vi "ROSTerminal.vi"() -> ()   [LabVIEW 2012]
doc: "Provides a space to debug any errors in code by:\n-allowing for testing connection to master\n-showing open nodes\n-linking to a website for viewing what is passed back and forth on a topic\n-linking to a website for the master to view what is passed back and forth\n-showing open logs\n-providing IP for you and Master"
uses:
  <userlib>/ROSforLV/ROS/Code/SubVIs/_ROSControl.ctl
  <userlib>/ROSforLV/ROS/Code/SubVIs/_ROSDirection.ctl
  <userlib>/ROSforLV/ROS/Code/_ROSDefinition.vi
  <vilib>/Platform/browser.llb/Open URL in Default Browser (string).vi
panel:
  out "elements":string[](array[string])
  in  "CloseServers":bool
  in  "Servers":i32(listbox)
  in  "Open HTML":bool
  in  "CloseNodes":bool
  in  "Nodes":i32(listbox)
  in  "ClearOldLogs":bool
  in  "Logs":i32(listbox)
  in  "OpenNodes":bool
  in  "MasterWeb":bool
  in  "MyWeb":bool
  in  "StartMaster":bool
  in  "UDP":bool
  out "My IP":string="http://192.168.1.8"
  in  "Done":bool
  out "Live":bool
  in  "Test":bool
  in  "Current Master":string="192.168.1.110:11311"
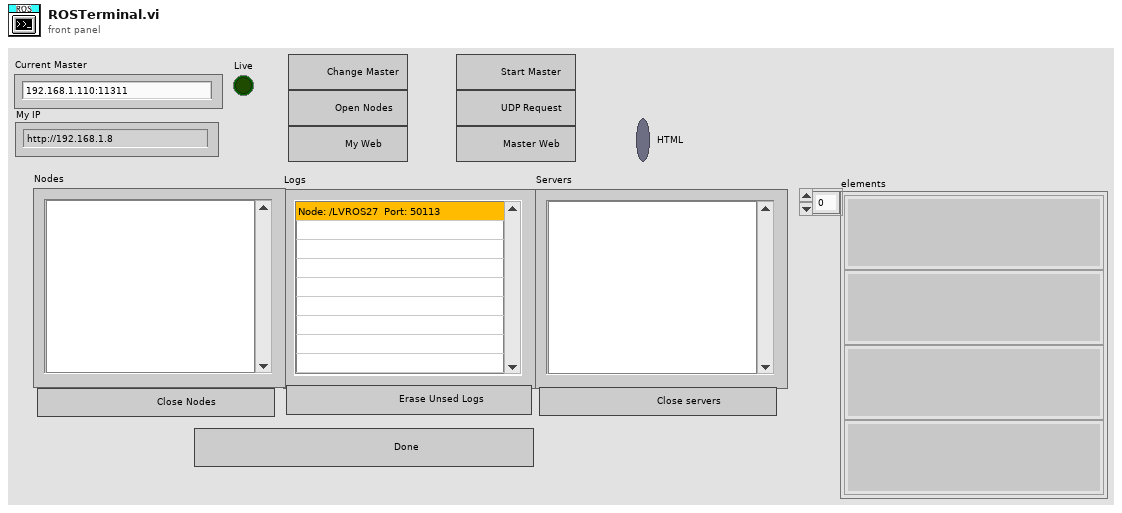
[diagram p1: front panel]
types:
  T1 = typedef "_ROSControl.ctl" = cluster{"topic port":u16, "Node":string, "topic":string, "type":string, "node port":u16, "error ":errorcluster, "Direction":T2, "Update (ms)":u16, "FIFO size":u16}
  T2 = typedef "_ROSDirection.ctl" = enum16{"Node", "Publisher", "Subscriber", "ServiceClient", "ServiceProvider"}
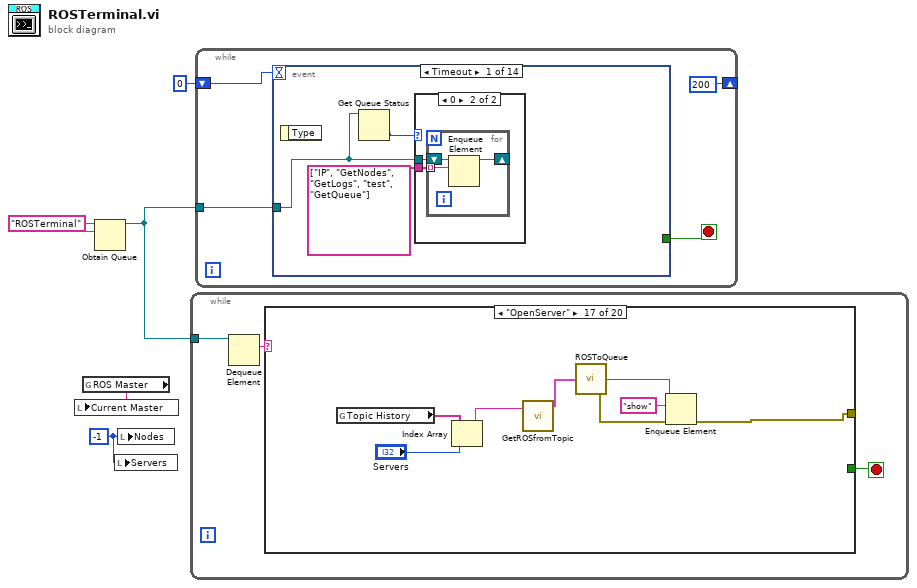
[diagram p0: block diagram]
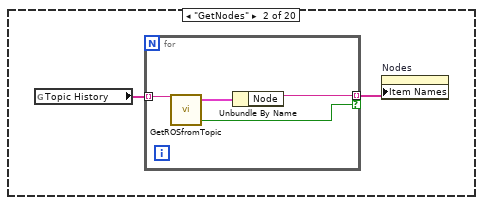
[diagram p3: hidden frame]
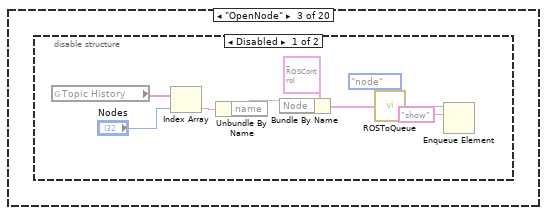
[diagram p4: hidden frame]
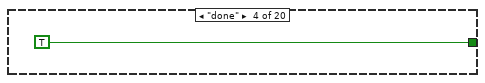
[diagram p6: hidden frame]
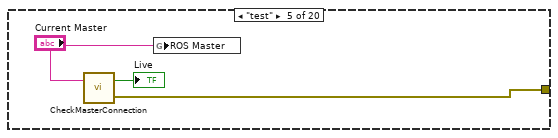
[diagram p7: hidden frame]
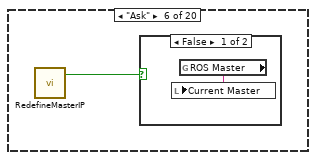
[diagram p8: hidden frame]
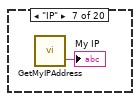
[diagram p10: hidden frame]
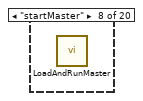
[diagram p11: hidden frame]
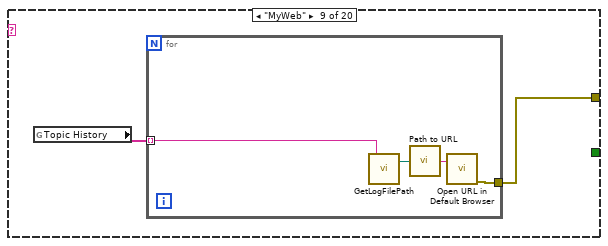
[diagram p12: hidden frame]
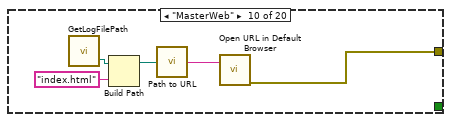
[diagram p13: hidden frame]
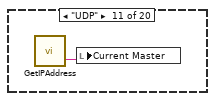
[diagram p14: hidden frame]
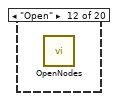
[diagram p15: hidden frame]
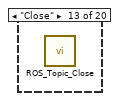
[diagram p16: hidden frame]
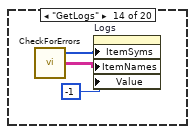
[diagram p17: hidden frame]
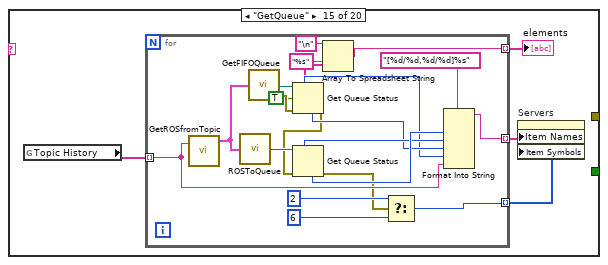
[diagram p18: hidden frame]
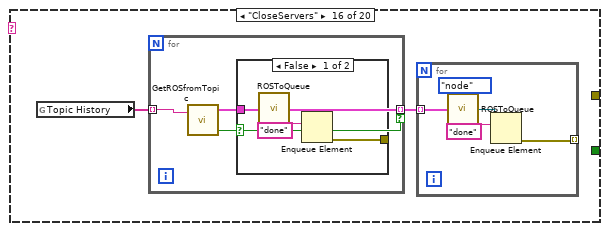
[diagram p19: hidden frame]
diagram:
  w1 = -1 ("Nodes")
  w4 = "ROSTerminal" ("name (unnamed)")
  n1 = global read "_ROSDefinition.vi" "ROS Master"() -> (w5:string)
  n2 = local write "Current Master"(w5) -> ()
  n3 = Obtain Queue(name (unnamed)=w4, element data type=w4) -> (queue out=w2:refnum<queue>)  [unwired: 3 in, 2 out]
  n4 = local write "Servers"(w1) -> ()
  n5 = local write "Nodes"(w1) -> ()
  n6 = while {
    tunnel: w2 -> [w8]
    stop <- w6 stop-if-true
    n7 = Dequeue Element(queue=w8) -> (element=w7:string)  [unwired: 2 in, 3 out]
    n8 = case shown="\"OpenServer\"" w7 {
      tunnel: [_ _ _ TRUE _ _ _ _ _ _ _ _ _ _ _ _ _ _ _ _] -> w6
      tunnel: [_ _ _ _ w25 _ _ _ w32 w37 _ _ _ _ _ _ w86 _ _ _] -> _
      frame Default {
      }
      frame "GetNodes" {
        n9 = global read "_ROSDefinition.vi" "Topic History"() -> (w10:string[])
        n10 = for {
          tunnel: w10 -> [w14] mode=indexing
          tunnel: [w11] -> w9 mode=indexing if=w12
          n11 = call <userlib>:"GetROSfromTopic.vi"("Topic"=w14) -> ("ROS"=w13:T1, "Node?"=w12:bool)  [unwired: 2 in]
          n12 = Unbundle By Name(w13) -> ("Node"=w11:string)
        }
        n13 = property on="Nodes" class="LstBox (strict)"("Item Names"=w9) -> ()  [unwired: 2 in, 2 out]
      }
      frame "OpenNode" {
        n14 = disable-structure shown="Disabled" {
          frame Disabled {
            n15 = global read "_ROSDefinition.vi" "Topic History"() -> (w23:string[])
            n16 = Index Array(array=w23, index="Nodes") -> (element=w21:string)
            n17 = Unbundle By Name(w21) -> ("name"=w15)
            n18 = Bundle By Name(cluster=T1 {"topic port"=0, "Node"="/fred", "topic"="/robot/head/command_head_nod", "type"="std_msgs/Bool", "node port"=59377, "error "={"status"=FALSE, "code"=0, "source"=""}, "Direction"=enum."Publisher", "Update (ms)"=1, "FIFO size"=1} ("ROS"), "Node"=w15) -> (w17:T1)
            n19 = call <userlib>:"ROSToQueue.vi"("ROS"=w17, "Name"=enum16{"topic", "node"}."node") -> ("queue"=w19:refnum<queue>)  [unwired: 2 in, 1 out]
            n20 = Enqueue Element(queue=w19, element="show") -> ()  [unwired: 2 in, 3 out]
          }
          frame Enabled {
          }
        }
      }
      frame "done" {
      }
      frame "test" {
        n21 = call <userlib>:"CheckMasterConnection.vi"("Master IP"="Current Master") -> ("error out"=w25:errorcluster, "Master There?"=→"Live":bool)  [unwired: 1 in]
        n22 = global write "_ROSDefinition.vi" "ROS Master"("Current Master") -> ()
      }
      frame "Ask" {
        n23 = call <userlib>:"RedefineMasterIP.vi"() -> ("Abort?"=w28:bool)  [unwired: 2 in]
        n24 = case shown="False" w28 {
          frame False {
            n25 = global read "_ROSDefinition.vi" "ROS Master"() -> (w29:string)
            n26 = local write "Current Master"(w29) -> ()
          }
          frame True {
          }
        }
      }
      frame "IP" {
        n27 = call <userlib>:"GetMyIPAddress.vi"() -> ("URI"=→"My IP":string)  [unwired: 2 in, 1 out]
      }
      frame "startMaster" {
        n28 = call <userlib>:"LoadAndRunMaster.vi"() -> ()  [unwired: 2 in, 2 out]
      }
      frame "MyWeb" {
        n29 = global read "_ROSDefinition.vi" "Topic History"() -> (w31:string[])
        n30 = for {
          tunnel: [w35] -> w32
          tunnel: w31 -> [w33] mode=indexing
          n31 = call <userlib>:"GetLogFilePath.vi"("Server name"=w33) -> ("LogPath"=w34:path)  [unwired: 1 in, 1 out]
          n32 = call <vilib>:"Path to URL.vi"("path"=w34) -> ("url"=w36:string)
          n33 = call-poly <vilib>:"Open URL in Default Browser.vi"("URL"=w36) -> ("error out"=w35:errorcluster)  [unwired: 5 in, 1 out]
        }
      }
      frame "MasterWeb" {
        n34 = call <userlib>:"GetLogFilePath.vi"() -> ("LogFolder"=w40:path)  [unwired: 2 in, 1 out]
        n35 = Build Path(base path=w40, name or relative path="index.html") -> (appended path=w38:path)
        n36 = call <vilib>:"Path to URL.vi"("path"=w38) -> ("url"=w41:string)
        n37 = call-poly <vilib>:"Open URL in Default Browser.vi"("URL"=w41) -> ("error out"=w37:errorcluster)  [unwired: 5 in, 1 out]
      }
      frame "UDP" {
        n38 = call <userlib>:"GetIPAddress.vi"() -> ("data out"=w42:string)  [unwired: 3 in]
        n39 = local write "Current Master"(w42) -> ()
      }
      frame "Open" {
        n40 = call <userlib>:"OpenNodes.vi"() -> ()  [unwired: 2 in]
      }
      frame "Close" {
        n41 = call <userlib>:"ROS_Topic_Close.vi"() -> ()  [unwired: 4 in, 1 out]
      }
      frame "GetLogs" {
        n42 = call <userlib>:"CheckForErrors.vi"() -> ("Symbols"=w44:i32[], "Logs"=w43:string[][])  [unwired: 2 in, 1 out]
        n43 = property on="Logs" class="MCListbox (strict)"("ItemSyms"=w44, "ItemNames"=w43, "Value"=-1 ("Listbox")) -> ()  [unwired: 2 in, 2 out]
      }
      frame "GetQueue" {
        n44 = global read "_ROSDefinition.vi" "Topic History"() -> (w49:string[])
        n45 = for {
          tunnel: w49 -> [w68] mode=indexing
          tunnel: [w70] -> w48 mode=indexing
          tunnel: [w69] -> w47 mode=indexing
          tunnel: [w50] -> w46 mode=indexing
          n46 = call <userlib>:"GetROSfromTopic.vi"("Topic"=w68) -> ("ROS"=w67:T1)  [unwired: 2 in, 1 out]
          n47 = call <userlib>:"ROSToQueue.vi"("ROS"=w67) -> ("queue"=w63:refnum<queue>)  [unwired: 3 in, 1 out]
          n48 = call <userlib>:"GetFIFOQueue.vi"("ROS"=w67) -> ("error out"=w57:errorcluster, "queue out"=w62:refnum<queue>)  [unwired: 3 in]
          n49 = Get Queue Status(queue=w62, return elements? (F)=TRUE, error in (no error)=w57) -> (max queue size=w58:i32, error out=w56:errorcluster, # elements in queue=w59:i32, elements=w53:string[])  [unwired: 4 out]
          n50 = Get Queue Status(queue=w63, error in (no error)=w56) -> (max queue size=w60:i32, error out=w55:errorcluster, # elements in queue=w61:i32)  [unwired: 1 in, 5 out]
          n51 = Array To Spreadsheet String(delimiter (Tab)="\n", array=w53, 3:"%s" ("format string")) -> (spreadsheet string=w50:string)
          n52 = Select(t=2, s=w55, f=6) -> (s? t:f=w69:i32)
          n53 = Format Into String(format string="[%d/%d,%d/%d]%s" ("name (unnamed)"), w61, w60, w59, w58, w68) -> (resulting string=w70:string)  [unwired: 2 in, 1 out]
        }
        "elements" <- w46
        n54 = property on="Servers" class="LstBox (strict)"("Item Names"=w48, "Item Symbols"=w47) -> ()  [unwired: 2 in, 2 out]
      }
      frame "CloseServers" {
        n55 = global read "_ROSDefinition.vi" "Topic History"() -> (w72:string[])
        n56 = for {
          tunnel: w72 -> [w80] mode=indexing
          tunnel: [w79] -> w71 mode=indexing if=w78
          n57 = call <userlib>:"GetROSfromTopic.vi"("Topic"=w80) -> ("ROS"=w79:T1, "Node?"=w78:bool)  [unwired: 2 in]
          n58 = case shown="False" w78 {
            tunnel: w79 -> [w83 _]
            tunnel: [w81 _] -> _
            frame False {
              n59 = call <userlib>:"ROSToQueue.vi"("ROS"=w83) -> ("queue"=w82:refnum<queue>)  [unwired: 3 in, 1 out]
              n60 = Enqueue Element(queue=w82, element="done") -> (error out=w81:errorcluster)  [unwired: 2 in, 2 out]
            }
            frame True {
            }
          }
        }
        n61 = for {
          tunnel: w71 -> [w75] mode=indexing
          tunnel: [w73] -> _ mode=indexing
          n62 = call <userlib>:"ROSToQueue.vi"("ROS"=w75, "Name"=enum16{"topic", "node"}."node") -> ("queue"=w77:refnum<queue>)  [unwired: 2 in, 1 out]
          n63 = Enqueue Element(queue=w77, element="done") -> (error out=w73:errorcluster)  [unwired: 2 in, 2 out]
        }
      }
      frame "OpenServer" {
        n64 = global read "_ROSDefinition.vi" "Topic History"() -> (w91:string[])
        n65 = Index Array(array=w91, index="Servers") -> (element=w89:string)
        n66 = call <userlib>:"GetROSfromTopic.vi"("Topic"=w89) -> ("ROS"=w87:T1)  [unwired: 2 in, 1 out]
        n67 = call <userlib>:"ROSToQueue.vi"("ROS"=w87) -> ("error out"=w85:errorcluster, "queue"=w88:refnum<queue>)  [unwired: 3 in]
        n68 = Enqueue Element(queue=w88, element="show", error in (no error)=w85) -> (error out=w86:errorcluster)  [unwired: 1 in, 2 out]
      }
      frame "OpenLogVI" {
        n69 = property on="Logs" class="MCListbox (strict)"() -> ("ItemNames"=w97:string[][], "Value"=w98:i32)  [unwired: 2 in, 2 out]
        n70 = Index Array(array=w97, index (row)=w98, index (col)=3 ("disabled index (col)")) -> (element=w102:string)
        n71 = Match Pattern(string=w102, regular expression="(") -> (before substring=w94:string, after substring=w103:string)  [unwired: 1 in, 2 out]
        n72 = Match Pattern(string=w103, regular expression=")") -> (before substring=w96:string, after substring=w105:string)  [unwired: 1 in, 2 out]
        n73 = call <vilib>:"Trim Whitespace.vi"("string"=w94) -> ("trimmed string"=w93:string)  [unwired: 1 in]
        n74 = call <vilib>:"Trim Whitespace.vi"("string"=w96) -> ("trimmed string"=w95:string)  [unwired: 1 in]
        n75 = case shown="\"Node\"" w105 {
          tunnel: T1 {"topic port"=0, "Node"="/fred", "topic"="/robot/head/command_head_nod", "type"="std_msgs/Bool", "node port"=59377, "error "={"status"=FALSE, "code"=0, "source"=""}, "Direction"=enum."Publisher", "Update (ms)"=1, "FIFO size"=1} ("ROS") -> [_ w114 w123 w132]
          tunnel: w93 -> [_ w108 w118 w127]
          tunnel: w95 -> [_ w107 w117 w126]
          tunnel: [_ w106 w115 w124] -> _
          frame Default {
          }
          frame "Publisher" {
            n76 = Bundle By Name(cluster=w114, "Node"=w107, "topic"=w108, "Direction"=_ROSDirection."Publisher") -> (w113:T1)
            n77 = call <userlib>:"ROSToQueue.vi"("ROS"=w113, "Name"=enum16{"topic", "node"}."topic") -> ("queue"=w111:refnum<queue>)  [unwired: 2 in, 1 out]
            n78 = Enqueue Element(queue=w111, element="show") -> (error out=w106:errorcluster)  [unwired: 2 in, 2 out]
          }
          frame "Subscriber" {
            n79 = Bundle By Name(cluster=w123, "Node"=w117, "topic"=w118, "Direction"=_ROSDirection."Subscriber") -> (w122:T1)
            n80 = call <userlib>:"ROSToQueue.vi"("ROS"=w122, "Name"=enum16{"topic", "node"}."topic") -> ("queue"=w120:refnum<queue>)  [unwired: 2 in, 1 out]
            n81 = Enqueue Element(queue=w120, element="show") -> (error out=w115:errorcluster)  [unwired: 2 in, 2 out]
          }
          frame "Node" {
            n82 = Bundle By Name(cluster=w132, "Node"=w126, "topic"=w127, "Direction"=_ROSDirection."Node") -> (w131:T1)
            n83 = call <userlib>:"ROSToQueue.vi"("ROS"=w131, "Name"=enum16{"topic", "node"}."node") -> ("queue"=w129:refnum<queue>)  [unwired: 2 in, 1 out]
            n84 = Enqueue Element(queue=w129, element="show") -> (error out=w124:errorcluster)  [unwired: 2 in, 2 out]
          }
        }
      }
      frame "OpenLogs" {
        n85 = property on="Logs" class="MCListbox (strict)"() -> ("ItemNames"=w137:string[][])  [unwired: 2 in, 2 out]
        n86 = Index Array(array=w137, index (row)="Logs") -> (element=w136:string[])  [unwired: 1 in]
        n87 = Index Array(array=w136, index=1) -> (element=w133:string)
        n88 = call-poly <vilib>:"Open URL in Default Browser.vi"("URL"=w133) -> ()  [unwired: 5 in, 2 out]
      }
      frame "EraseLogs" {
        n89 = call <userlib>:"CheckForErrors.vi"() -> ("Symbols"=w139:i32[], "Paths"=w138:path[])  [unwired: 2 in, 1 out]
        n90 = for {
          tunnel: w139 -> [w141] mode=indexing
          tunnel: w138 -> [w140] mode=indexing
          n91 = case shown="0" w141 {
            tunnel: [w143 _] -> _
            tunnel: w140 -> [w142 _]
            frame 0 {
              n92 = Delete(path (use dialog)=w142) -> (error out=w143:errorcluster)  [unwired: 4 in, 2 out]
            }
            frame Default {
            }
          }
        }
      }
    }
  }
  n93 = while {
    tunnel: w2 -> [w147]
    shift-right: [200 ("timeout in ms (-1)")] -> _
    shift-left: 0 ("timeout in ms (-1)") -> [w144]
    stop <- w146 stop-if-true
    n94 = event shown="[0] Timeout" {
      selector: _ -> [_ _ _ _ _ _ _ _ _ _ _ _ _ _]
      dyn-events: _ -> [_ _ _ _ _ _ _ _ _ _ _ _ _ _]
      timeout: w144 -> [_ _ _ _ _ _ _ _ _ _ _ _ _ _]
      tunnel: w147 -> [w149 w157 w159 w161 w163 w169 w171 w173 w175 w179 w181 w183 w185 w188]
      tunnel: [_ _ _ _ _ _ _ _ _ _ _ _ _ "Done"] -> w146
      event Timeout {
        n95 = event-data() -> ()  [unwired: 1 in, 1 out]
        n96 = Get Queue Status(queue=w149) -> (# elements in queue=w148:i32)  [unwired: 2 in, 7 out]
        n97 = case shown="0" w148 {
          tunnel: string[] ["IP", "GetNodes", "GetLogs", "test", "GetQueue"] -> [_ w152]
          tunnel: w149 -> [_ w151]
          frame Default {
          }
          frame 0 {
            n98 = for {
              shift-right: [w155] -> _
              shift-left: w151 -> [w154]
              tunnel: w152 -> [w153] mode=indexing
              n99 = Enqueue Element(queue=w154, element=w153) -> (queue out=w155:refnum<queue>)  [unwired: 2 in, 2 out]
            }
          }
        }
      }
      event "Test", "Current Master": Value Change {
        n100 = event-data() -> ()  [unwired: 1 in, 1 out]
        n101 = Enqueue Element(queue=w157, element="Ask") -> ()  [unwired: 2 in, 3 out]
      }
      event "StartMaster": Value Change {
        n102 = event-data() -> ()  [unwired: 1 in, 1 out]
        n103 = Enqueue Element(queue=w159, element="startMaster") -> ()  [unwired: 2 in, 3 out]
      }
      event "MyWeb": Value Change {
        n104 = event-data() -> ()  [unwired: 1 in, 1 out]
        n105 = Enqueue Element(queue=w161, element="MyWeb") -> ()  [unwired: 2 in, 3 out]
      }
      event "UDP": Value Change {
        n106 = event-data() -> ()  [unwired: 1 in, 1 out]
        n107 = Enqueue Element(queue=w163, element="UDP") -> ()  [unwired: 2 in, 3 out]
      }
      event "Logs": Value Change {
        n108 = event-data() -> ()  [unwired: 1 in, 1 out]
        n109 = Not(x="Open HTML") -> (.not. x?=w164:bool)
        n110 = Select(t="OpenLogs" ("element"), s=w164, f="OpenLogVI" ("element")) -> (s? t:f=w165:string)
        n111 = Enqueue Element(queue=w169, element=w165) -> ()  [unwired: 2 in, 3 out]
      }
      event "Servers": Value Change; "Servers": Double Click {
        n112 = event-data() -> ()  [unwired: 1 in, 3 out]
        n113 = Enqueue Element(queue=w171, element="OpenServer") -> ()  [unwired: 2 in, 3 out]
      }
      event "CloseServers": Value Change {
        n114 = event-data() -> ()  [unwired: 1 in, 5 out]
        n115 = Enqueue Element(queue=w173, element="CloseServers") -> ()  [unwired: 2 in, 3 out]
      }
      event "Nodes": Value Change {
        n116 = event-data() -> ()  [unwired: 1 in, 5 out]
        n117 = Enqueue Element(queue=w175, element="OpenNode") -> ()  [unwired: 2 in, 3 out]
      }
      event "ClearOldLogs": Value Change {
        n118 = event-data() -> ()  [unwired: 1 in, 5 out]
        n119 = Enqueue Element(queue=w179, element="EraseLogs") -> (queue out=w177:refnum<queue>)  [unwired: 2 in, 2 out]
        n120 = Enqueue Element(queue=w177, element="GetLogs") -> ()  [unwired: 2 in, 3 out]
      }
      event "OpenNodes": Value Change {
        n121 = event-data() -> ()  [unwired: 1 in, 1 out]
        n122 = Enqueue Element(queue=w181, element="Open") -> ()  [unwired: 2 in, 3 out]
      }
      event "CloseNodes": Value Change {
        n123 = event-data() -> ()  [unwired: 1 in, 1 out]
        n124 = Enqueue Element(queue=w183, element="Close") -> ()  [unwired: 2 in, 3 out]
      }
      event "MasterWeb": Value Change {
        n125 = event-data() -> ()  [unwired: 1 in, 1 out]
        n126 = Enqueue Element(queue=w185, element="MasterWeb") -> ()  [unwired: 2 in, 3 out]
      }
      event "Done": Value Change {
        n127 = event-data() -> ()  [unwired: 1 in, 1 out]
        n128 = Enqueue Element(queue=w188, element="done") -> ()  [unwired: 2 in, 3 out]
      }
    }
  }
